vi "test_MultipleSessionsReserved_CallCreateSessions_SessionsAddedToCollectionMap.vi"(8 "error in":errorcluster) -> (0 "error out":errorcluster, 2 "result":string, 3 "pass":bool)   [LabVIEW 2020, in "MeasurementServerTests.lvlib"]
uses:
  MeasurementServerTests.lvlib
  Runtime/MeasurementLink Session Management/Session Reservation/Connection with Session.ctl
  Runtime/MeasurementLink Session Management/Session Reservation/Connection.ctl
  ae719597-ef3c-4b10-9a49-a4238caa881c.vi
  69564c08-2d8d-4b91-a54b-51eac17b37e1.vi
  da6ffb6f-c1c9-4957-84dd-e9228483c454.vi
  a956f7ee-c7e9-4639-884c-f4265dae6ecf.vi
  5728b933-7d39-4da4-b754-5b48616fa0f3.vi
  Helpers/Fake Instrument/Fake Instrument.lvclass
  C:/dev/measurementlink-labview/Source/Runtime/MeasurementLink Instrument/IInstrument/IInstrument.lvclass
  Runtime/MeasurementLink Session Management/Session Reservation/Create Sessions Dispatcher.vi
  Runtime/MeasurementLink Session Management/Session Reservation/Get Connections Dispatcher.vi
  Runtime/MeasurementLink Session Management/Session Reservation/Session Reservation.lvclass
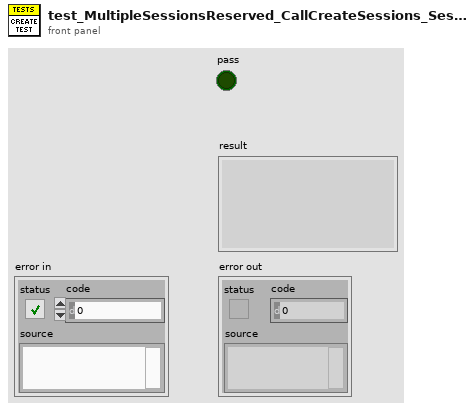
[diagram p1: front panel]
types:
  T1 = typedef "MeasurementLink Session Management.lvlib/Session Reservation.lvclass/Connection.ctl" = cluster{"pin or relay name":string, "site":i32, "instrument type id":string, "channel":string}
  T2 = typedef "MeasurementLink Session Management.lvlib/Session Reservation.lvclass/Connection with Session.ctl" = cluster{"connection":T1, "session":variant}
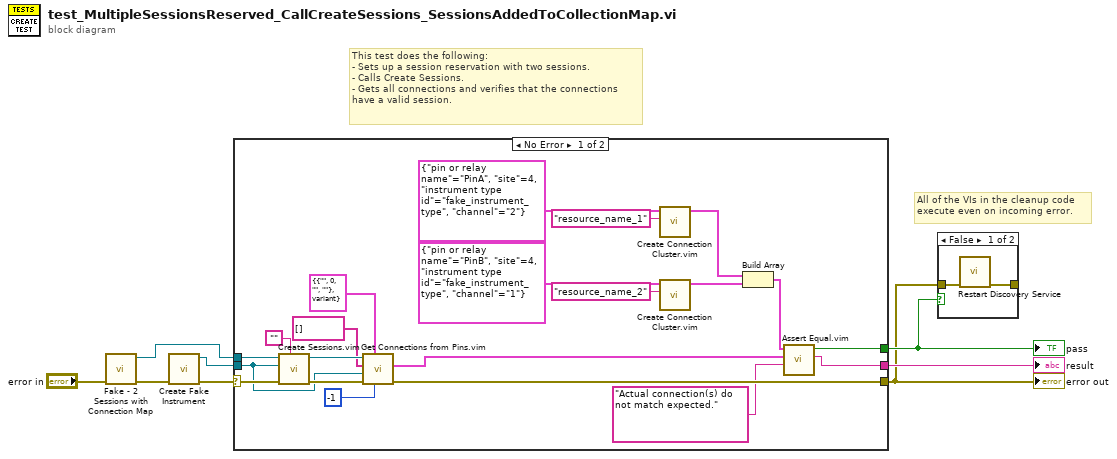
[diagram p0: block diagram]
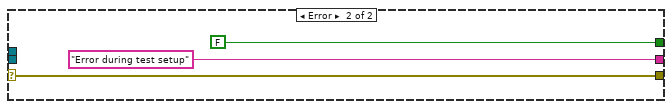
[diagram p2: hidden frame]
diagram:
  # "All of the VIs in the cleanup code\nexecute even on incoming error."
  # "This test does the following:\n- Sets up a session reservation with two sessions.\n- Calls Create Sessions.\n- Gets all connections and verifies that the connections\nhave a valid session."
  n1 = call "Fake - 2 Sessions with Connection Map.vi"("error in"="error in") -> ("error out"=w2:errorcluster, "session reservation out"=w1:refnum<class "Session Reservation.lvclass">)  [unwired: 9 in]
  n2 = call "Create Fake Instrument.vi"("error in"=w2) -> ("error out"=w5:errorcluster, "fake instrument out"=w4:refnum<class "Fake Instrument.lvclass">)  [unwired: 9 in]
  n3 = case shown="No Error" w5 {
    selector: w5 -> [w28 w30]
    tunnel: [w18 w30] -> w6
    tunnel: [w20 FALSE] -> w7
    tunnel: [w19 "Error during test setup" ("f")] -> w8
    tunnel: w4 -> [w23 _]
    tunnel: w1 -> [w29 _]
    frame No Error {
      n4 = call "Create Sessions.vim"("session type"="", "error in"=w28, "instrument"=w23, "session reservation in"=w29) -> ("error out"=w26:errorcluster, "session reservation out"=w25:refnum<class "Session Reservation.lvclass">)  [unwired: 4 in, 2 out]
      n5 = call "Get Connections from Pins.vim"("site"=-1, "connection type"=T2 {"connection"={"pin or relay name"="", "site"=0, "instrument type id"="", "channel"=""}, "session"=variant}, "error in"=w26, "instrument"=w23, "pin or relay names"=string[] [], "session reservation in"=w25) -> ("error out"=w18:errorcluster, "connections"=w17:T2[])  [unwired: 3 in, 1 out]
      n6 = call "Create Connection Cluster.vim"("session in"="resource_name_1", "hardware independent connection in"=T1 {"pin or relay name"="PinA", "site"=4, "instrument type id"="fake_instrument_type", "channel"="2"} ("connection")) -> ("connection out"=w14:T2)  [unwired: 9 in]
      n7 = call "Create Connection Cluster.vim"("session in"="resource_name_2", "hardware independent connection in"=T1 {"pin or relay name"="PinB", "site"=4, "instrument type id"="fake_instrument_type", "channel"="1"} ("connection")) -> ("connection out"=w13:T2)  [unwired: 9 in]
      n8 = Build Array(w14, w13) -> (w12:T2[])
      n9 = call "Assert Equal.vim"("failure message"="Actual connection(s) do not match expected.", "actual value"=w17, "expected value"=w12) -> ("message"=w19:string, "equal?"=w20:bool)  [unwired: 7 in]
    }
    frame Error {
    }
  }
  "error out" <- w6
  "pass" <- w7
  "result" <- w8
  n10 = case shown="False" w7 {
    tunnel: w6 -> [w34 _]
    tunnel: [w33 _] -> _
    frame False {
      n11 = call "Restart Discovery Service.vi"("error in"=w34) -> ("error out"=w33:errorcluster)  [unwired: 10 in]
    }
    frame True {
    }
  }
